vi "TurnInPlace.vi"(9 "Angle Setpoint":dbl) -> ()   [LabVIEW 2016, in "DriveBase.lvclass"]
uses:
  DriveBase.lvclass
  DriveStates.ctl
  <vilib>/addons/control/pid/pid.llb/PID (DBL).vi
  <vilib>/addons/control/pid/NI_PID_pid.lvlib
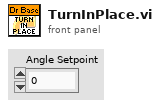
[diagram p1: front panel]
types:
  T1 = typedef "DriveBase.lvclass/DriveStates.ctl" = enum16{"Tank", "Arcade", "DriveStraight"}
  T2 = cluster{"proportional gain (Kc)":dbl, "integral time (Ti, min)":dbl, "derivative time (Td, min)":dbl}
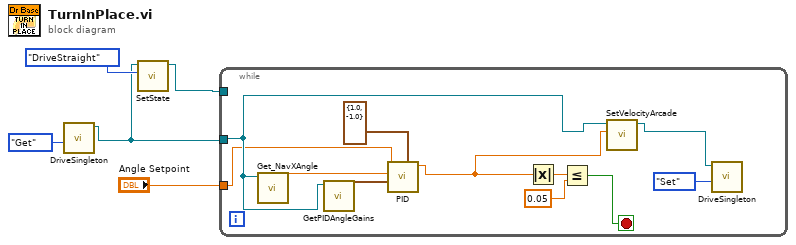
[diagram p0: block diagram]
diagram:
  n1 = call "DriveSingleton.vi"("Get/Set"=enum16{"Get", "Set"}."Get") -> ("DriveBase.lvclass 2"=w2:refnum<class "DriveBase.lvclass">)  [unwired: 9 in, 1 out]
  n2 = call-dynamic "SetState.vi"("State"=DriveStates."DriveStraight", "DriveBase in"=w2) -> ("DriveBase out"=w1:refnum<class "DriveBase.lvclass">)  [unwired: 8 in, 1 out]
  n3 = while {
    tunnel: w2 -> [w10]
    tunnel: "Angle Setpoint" -> [w8]
    tunnel: w1 -> [_]
    stop <- w11 stop-if-true
    n4 = call-dynamic "Get_NavXAngle.vi"("DriveBase in"=w10) -> ("NavX Angle"=w16:dbl)  [unwired: 9 in, 1 out]
    n5 = call "GetPIDAngleGains.vi"("DriveBase.lvclass"=w10) -> ("Angle PID gains"=w15:T2)  [unwired: 9 in, 1 out]
    n6 = call-poly <vilib>:"PID.vi"("output range"=cluster{"output high":dbl, "output low":dbl} {"output high"=1.0, "output low"=-1.0}, "PID gains"=w15, "process variable"=w16, "setpoint"=w8) -> ("output"=w9:dbl)  [unwired: 6 in, 1 out]
    n7 = Absolute Value(x=w9) -> (abs(x)=w13:dbl)
    n8 = Less Or Equal?(x=w13, y=0.05) -> (x <= y?=w11:bool)
    n9 = call "SetVelocityArcade.vi"("X Axis"=w9, "DriveBase.lvclass"=w10) -> ("DriveBase.lvclass"=w6:refnum<class "DriveBase.lvclass">)  [unwired: 8 in, 1 out]
    n10 = call "DriveSingleton.vi"("Get/Set"=enum16{"Get", "Set"}."Set", "DriveBase.lvclass"=w6) -> ()  [unwired: 8 in, 2 out]
  }
